vi "flash.vi"() -> ()   [LabVIEW 2022 SP3]
uses:
  Program Files/National Instruments/LabVIEW 2024/user.lib/pcanbasic/constants/PCAN Bitrates.ctl
  Program Files/National Instruments/LabVIEW 2024/user.lib/pcanbasic/constants/PCAN Devices.ctl
  Program Files/National Instruments/LabVIEW 2024/user.lib/pcanbasic/PCANBasic.lvlib
panel:
  out "Progress":u8(slide) scale=0.0..100.0
  in  "OK Button":bool
  out "CRC32Value":u32 format="%x"
  out "Payload Size (Bytes)":i32
  in  "Firmware Path":path
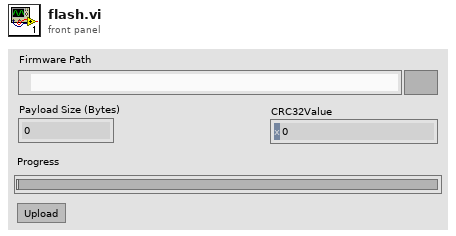
[diagram p1: front panel]
types:
  T1 = typedef "PCANBasic.lvlib/PCAN Devices.ctl" = enum8{"PCAN_NONE", "PCAN_PEAKCAN", "PCAN_ISA", "PCAN_DNG", "PCAN_PCI", "PCAN_USB", "PCAN_PCC", "PCAN_VIRTUAL", "PCAN_LAN"}
  T2 = cluster{"ID":u32, "MSGTYPE":u8, "LEN":u8, "DATA[0]":u8, "DATA[1]":u8, "DATA[2]":u8, "DATA[3]":u8, "DATA[4]":u8, "DATA[5]":u8, "DATA[6]":u8, "DATA[7]":u8}
  T3 = typedef "PCANBasic.lvlib/PCAN Bitrates.ctl" = u16
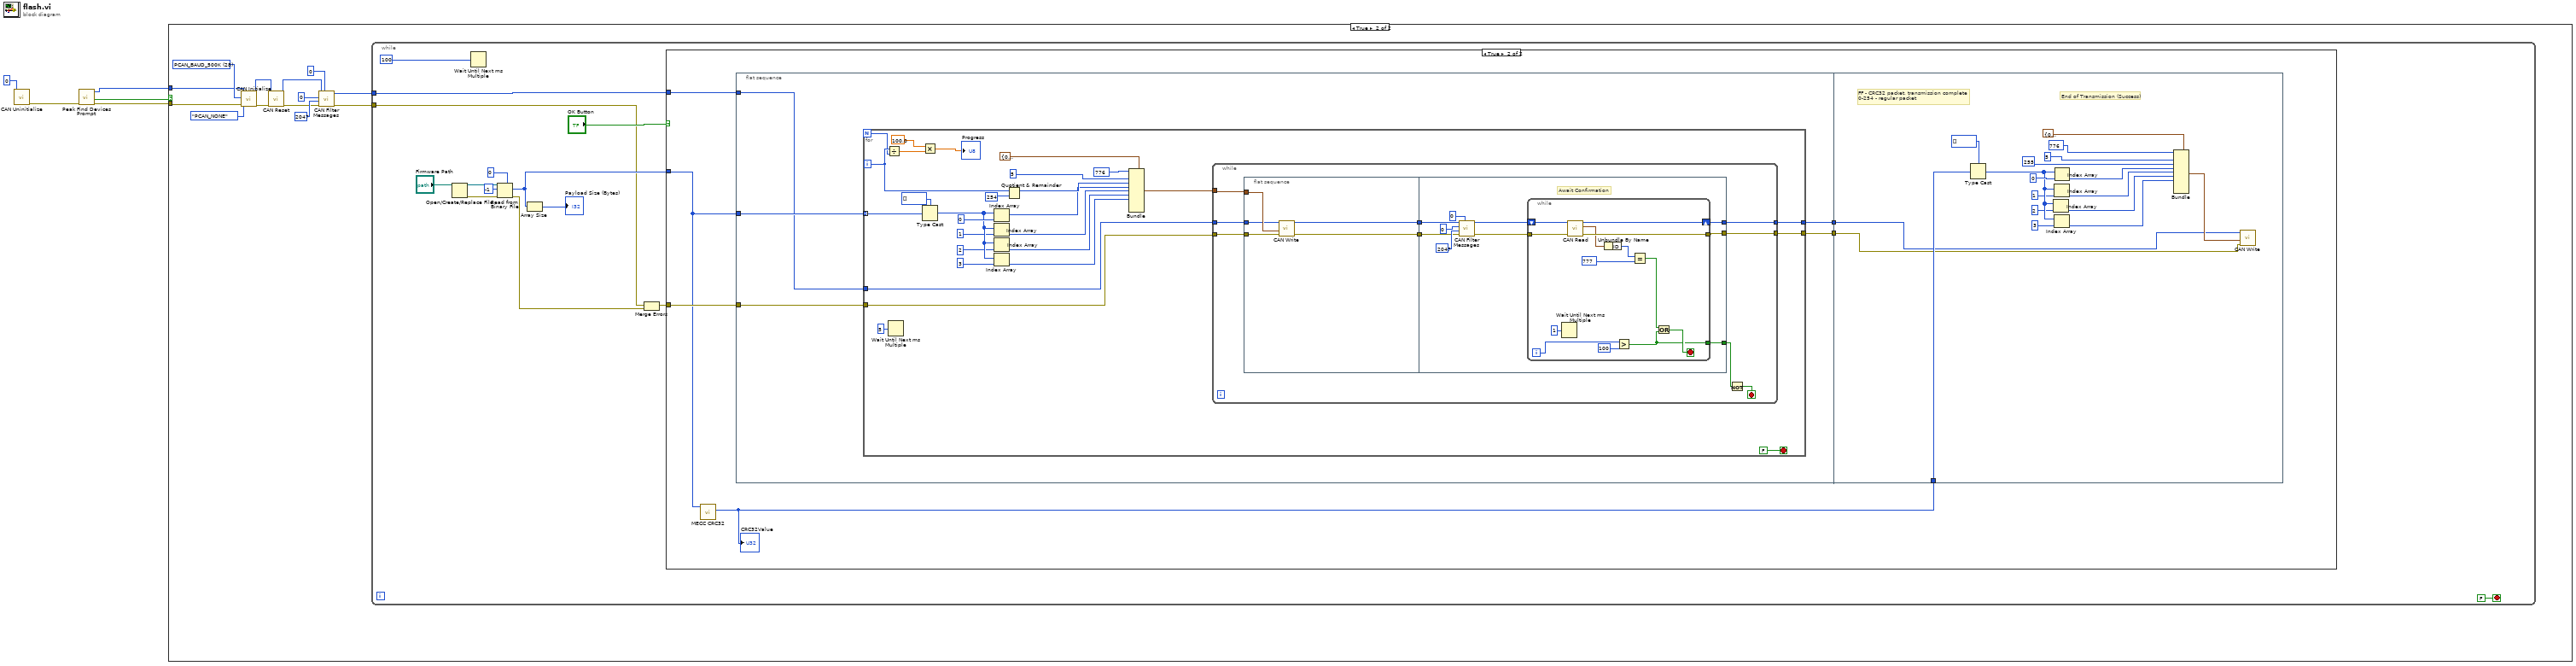
[diagram p0: block diagram]
diagram:
  n1 = call "CAN Uninitialize.vi"("Channel"=u16 0) -> ("error out"=w2:errorcluster)  [unwired: 9 in, 1 out]
  n2 = call "Peak Find Devices Prompt.vi"("error in (no error)"=w2) -> ("error out"=w4:errorcluster, "Found?"=w3:bool, "CAN Channel"=w5:u16)  [unwired: 8 in]
  n3 = case shown="True" w3 {
    tunnel: w5 -> [_ w8]
    tunnel: w4 -> [_ w7]
    frame False {
    }
    frame True {
      w17 = T3 28 items=["PCAN_BAUD_1M"=20, "PCAN_BAUD_800K"=22, "PCAN_BAUD_500K"=28, "PCAN_BAUD_250K "=284, "PCAN_BAUD_125K "=796, "PCAN_BAUD_100K"=17199, "PCAN_BAUD_95K"=49998, "PCAN_BAUD_83K"=34091, "PCAN_BAUD_50K"=18223, "PCAN_BAUD_47K"=5140, "PCAN_BAUD_33K"=35631, "PCAN_BAUD_20K"=21295, "PCAN_BAUD_10K"=26415, "PCAN_BAUD_5K"=32639] ("PCAN Baud rate")
      n4 = call "CAN Initialize.vi"("error in (no error)"=w7, "PCAN Devices"=PCAN_Devices."PCAN_NONE", "PCAN Baud rate"=w17, "Channel"=w8) -> ("error out"=w14:errorcluster, "Channel Out"=w15:u16)  [unwired: 5 in, 1 out]
      n5 = call "CAN Reset.vi"("error in (no error)"=w14, "Channel"=w15) -> ("error out"=w10:errorcluster, "Channel Out"=w13:u16)  [unwired: 7 in, 1 out]
      n6 = call "CAN Filter Messages.vi"("Mode"=u8 0, "error in (no error)"=w10, "ToID"=u32 2047, "FromID"=u32 0, "Channel"=w13) -> ("error out"=w18:errorcluster, "Channel Out"=w6:u16)  [unwired: 4 in, 1 out]
      n7 = while {
        tunnel: w18 -> [w20]
        tunnel: w6 -> [w22]
        stop <- FALSE stop-if-true
        n8 = Open/Create/Replace File(file path (use dialog)="Firmware Path") -> (refnum out=w29:refnum<file>, error out=w28:errorcluster)  [unwired: 5 in, 1 out]
        n9 = Wait Until Next ms Multiple(millisecond multiple=u32 100) -> ()  [unwired: 1 out]
        n10 = Read from Binary File(5:u32 0, 8:w28, 10:-1 ("count (1)"), 11:w29) -> (0:w19:errorcluster, 2:w25:u32[])  [unwired: 2 in, 2 out]
        n11 = Array Size(array=w25) -> (size(s)=→"Payload Size (Bytes)":i32)
        n12 = Merge Errors(w20, w19) -> (w21:errorcluster)
        n13 = case shown="True" "OK Button" {
          tunnel: w21 -> [_ w38]
          tunnel: w25 -> [_ w35]
          tunnel: w22 -> [_ w34]
          frame False {
          }
          frame True {
            n14 = call "MECC CRC32.vi"("Data"=w35) -> ("CRC32Value"=w33:u32)  [unwired: 10 in]
            "CRC32Value" <- w33
            n15 = flat-sequence {
              tunnel: w38 -> [w43]
              tunnel: [w42] -> w37
              tunnel: [w41] -> w36
              tunnel: w35 -> [w40]
              tunnel: w34 -> [w39]
              tunnel: w33 -> [w117]
              tunnel: w37 -> [w115]
              tunnel: w36 -> [w114]
              frame #0 {
                n16 = for {
                  N -> [w48]
                  tunnel: w40 -> [w63] mode=indexing
                  tunnel: w43 -> [w65]
                  tunnel: [w56] -> w42
                  tunnel: [w46] -> w41
                  tunnel: w39 -> [w44]
                  i -> [w49]
                  stop <- FALSE stop-if-true
                  n17 = Divide(x=w49, y=w48) -> (x/y=w71:dbl)
                  n18 = Wait Until Next ms Multiple(millisecond multiple=u32 5) -> ()  [unwired: 1 out]
                  n19 = Multiply(x=100.0, y=w71) -> (x*y=→"Progress":dbl)
                  n20 = Type Cast(type=u8[] [], x=w63) -> (*(type *) &x=w60:u8[])
                  n21 = Index Array(array=w60, index=1) -> (element=w52:u8)
                  n22 = Index Array(array=w60, index=3) -> (element=w50:u8)
                  n23 = Index Array(array=w60, index=0) -> (element=w53:u8)
                  n24 = Index Array(array=w60, index=2) -> (element=w51:u8)
                  n25 = Quotient & Remainder(x=w49, y=254) -> (x-y*floor(x/y)=w54:i32)  [unwired: 1 out]
                  n26 = Bundle(cluster=T2 {"ID"=0, "MSGTYPE"=0, "LEN"=0, "DATA[0]"=0, "DATA[1]"=0, "DATA[2]"=0, "DATA[3]"=0, "DATA[4]"=0, "DATA[5]"=0, "DATA[6]"=0, "DATA[7]"=0} ("MessageBuffer"), "ID"=u32 776, "LEN"=u8 5, "DATA[0]"=w54, "DATA[1]"=w53, "DATA[2]"=w52, "DATA[3]"=w51, "DATA[4]"=w50) -> (w66:T2)  [unwired: 4 in]
                  n27 = while {
                    tunnel: w66 -> [w77]
                    tunnel: w65 -> [w76]
                    tunnel: [w72] -> w46
                    tunnel: w44 -> [w78]
                    tunnel: [w75] -> w56
                    stop <- w73 stop-if-true
                    n28 = flat-sequence {
                      tunnel: w78 -> [w81]
                      tunnel: w77 -> [w85]
                      tunnel: w76 -> [w84]
                      tunnel: [w83] -> w80
                      tunnel: [w82] -> w79
                      tunnel: [w95] -> w75
                      tunnel: w80 -> [w91]
                      tunnel: w79 -> [w89]
                      tunnel: [w87] -> w74
                      tunnel: [w86] -> w72
                      frame #0 {
                        n29 = call "CAN Write.vi"("error in (no error)"=w84, "MessageBuffer"=w85, "Channel"=w81) -> ("error out"=w82:errorcluster, "Channel Out"=w83:u16)  [unwired: 5 in, 2 out]
                      }
                      frame #1 {
                        # "Await Confirmation"
                        n30 = call "CAN Filter Messages.vi"("Mode"=u8 0, "error in (no error)"=w89, "ToID"=u32 2047, "FromID"=u32 0, "Channel"=w91) -> ("error out"=w88:errorcluster, "Channel Out"=w90:u16)  [unwired: 4 in, 1 out]
                        n31 = while {
                          shift-right: [w108] -> w95
                          shift-left: w90 -> [w107]
                          tunnel: w88 -> [w106]
                          tunnel: [w105] -> w86
                          tunnel: [w96] -> w87
                          i -> [w100]
                          stop <- w97 stop-if-true
                          n32 = Wait Until Next ms Multiple(millisecond multiple=u32 1) -> ()  [unwired: 1 out]
                          n33 = call "CAN Read.vi"("error in (no error)"=w106, "Channel"=w107) -> ("error out"=w105:errorcluster, "MessageBuffer out"=w103:T2, "Channel Out"=w108:u16)  [unwired: 5 in, 2 out]
                          n34 = Unbundle By Name(w103) -> ("ID"=w102:u32)
                          n35 = Greater?(x=w100, y=100) -> (0:w96:bool)
                          n36 = Equal?(x=w102, y=u32 777) -> (x = y?=w98:bool)
                          n37 = Or(x=w98, y=w96) -> (x .or. y?=w97:bool)
                        }
                      }
                    }
                    n38 = Not(x=w74) -> (.not. x?=w73:bool)
                  }
                }
              }
              frame #1 {
                # "FF - CRC32 packet, transmission complete\n0-254 - regular packet"
                # "End of Transmission (Success)"
                n39 = Type Cast(type=u8[] [], x=w117) -> (*(type *) &x=w121:u8[])
                n40 = Index Array(array=w121, index=2) -> (element=w110:u8)
                n41 = Index Array(array=w121, index=1) -> (element=w111:u8)
                n42 = Index Array(array=w121, index=3) -> (element=w109:u8)
                n43 = Index Array(array=w121, index=0) -> (element=w112:u8)
                n44 = Bundle(cluster=T2 {"ID"=0, "MSGTYPE"=0, "LEN"=0, "DATA[0]"=0, "DATA[1]"=0, "DATA[2]"=0, "DATA[3]"=0, "DATA[4]"=0, "DATA[5]"=0, "DATA[6]"=0, "DATA[7]"=0} ("MessageBuffer"), "ID"=u32 776, "LEN"=u8 5, "DATA[0]"=u8 255, "DATA[1]"=w112, "DATA[2]"=w111, "DATA[3]"=w110, "DATA[4]"=w109) -> (w116:T2)  [unwired: 4 in]
                n45 = call "CAN Write.vi"("error in (no error)"=w114, "MessageBuffer"=w116, "Channel"=w115) -> ()  [unwired: 5 in, 4 out]
              }
            }
          }
        }
      }
    }
  }
